vi "GUI_001.vi"(2 "Input":dbl) -> (0 "Slide":dbl(slide) scale=0.0..100.0)   [LabVIEW 2022 SP3]
panel:
  in  "Gain":dbl
  in  "Offset":dbl
  in  "Enum":enum16{"Manual", "Random"}(ring)
  out "Waveform Chart":dbl(graph)
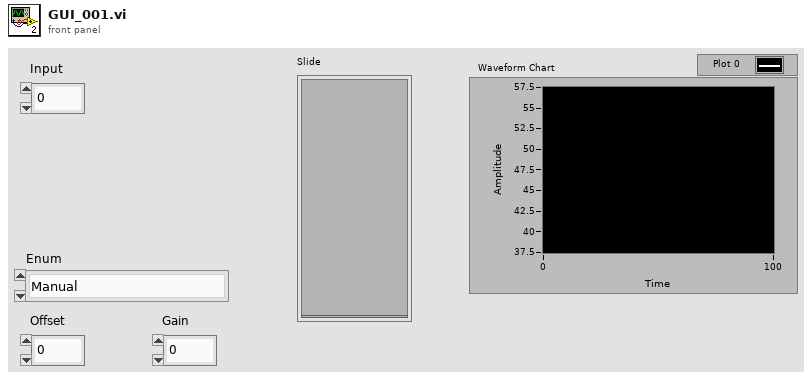
[diagram p1: front panel]
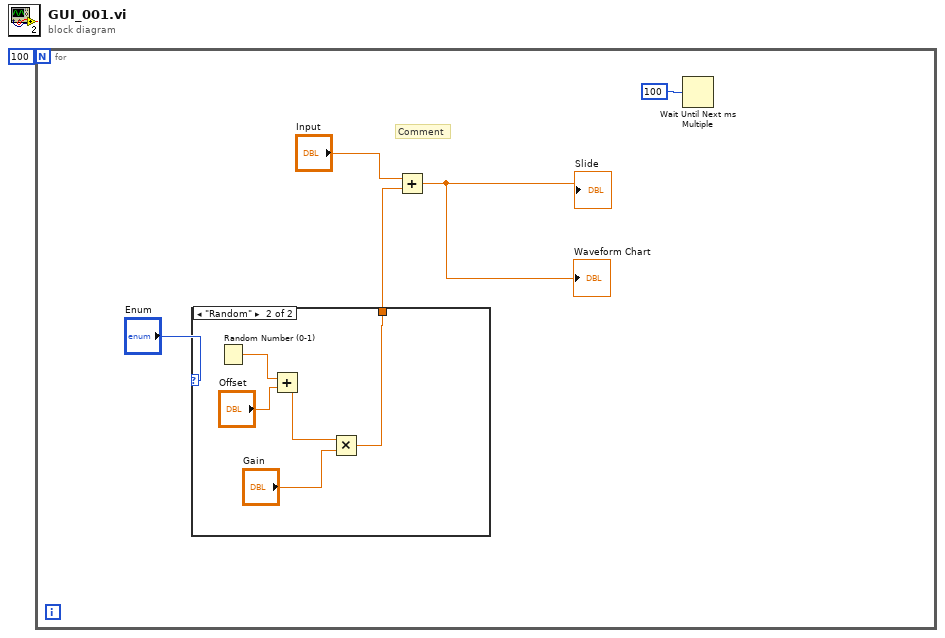
[diagram p0: block diagram]
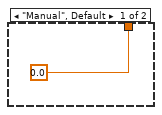
[diagram p2: hidden frame]
diagram:
  n1 = for {
    N: 100 -> [_]
    # "Comment"
    n2 = case shown="\"Random\"" "Enum" {
      tunnel: [0.0 w12] -> w2
      frame "Manual", Default {
      }
      frame "Random" {
        n3 = Random Number (0-1)() -> (number: 0 to 1=w11:dbl)
        n4 = Add(x=w11, y="Offset") -> (x+y=w10:dbl)
        n5 = Multiply(x=w10, y="Gain") -> (x*y=w12:dbl)
      }
    }
    n6 = Add(x="Input", y=w2) -> (x+y=→"Slide" →"Waveform Chart":dbl)
    n7 = Wait Until Next ms Multiple(millisecond multiple=u32 100) -> ()  [unwired: 1 out]
  }
